vi "Get Data.vi"(8 "error in":errorcluster, 11 "Airmar WS in":refnum<class "Airmar WS.lvclass">) -> (0 "error out":errorcluster, 2 "Data":refnum<class "Data.lvclass">, 3 "Airmar WS out":refnum<class "Airmar WS.lvclass">)   [LabVIEW 2014, in "Airmar WS.lvclass"]
uses:
  Airmar WS.lvclass
  Reusable/Session APIs/Text Communication/Text Device Session.lvclass
  Data/Airmar Data.lvclass
  Reusable/Data/Data.lvclass
panel:
  out "Data":string
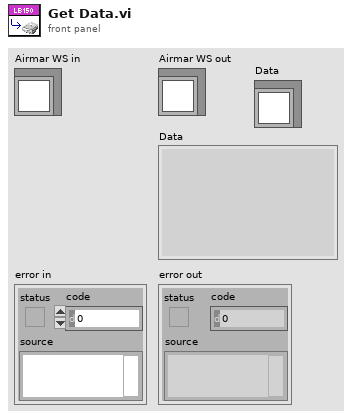
[diagram p1: front panel]
types:
  T1 = typedef "Session - Root.lvclass/Session Handle.ctl" = refnum<data-value>
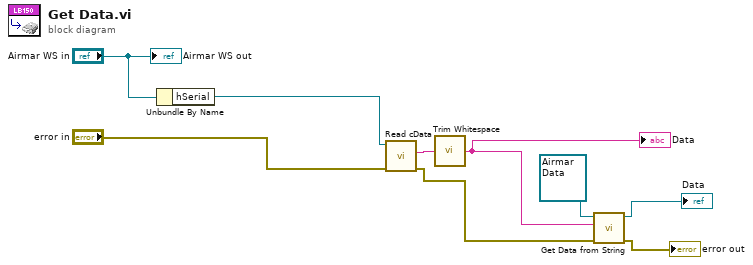
[diagram p0: block diagram]
diagram:
  n1 = Unbundle By Name("Airmar WS in") -> ("hSerial"=w8:T1)
  n2 = call "Read cData.vi"("error in"="error in", "hSession In"=w8) -> ("error out"=w5:errorcluster, "Data"=w7:string)  [unwired: 7 in, 1 out]
  n3 = call <vilib>:"Trim Whitespace.vi"("string"=w7) -> ("trimmed string"=w4:string)  [unwired: 1 in]
  "Data" <- w4
  n4 = call "Get Data from String.vi"("error in (no error)"=w5, "DataIn"=w4, "Airmar Data in"=refnum<class "Airmar Data.lvclass"> refnum) -> ("error out"=→"error out":errorcluster, "Airmar Data out"=→"Data":refnum<class "Airmar Data.lvclass">)  [unwired: 7 in]
  "Airmar WS out" <- "Airmar WS in"
